vi "Pump Tags.vi"(11 "Pump Module Configs":T1[](array[typedef]) {"Settings"."ASIA Pump C"."channel" min=0 max=1 step=1; "Settings"."Masterflex"."Pump Number" min=1.0 max=20.0 step=1.0; "Settings"."Ismatech"."Pump Number" min=1.0 max=20.0 step=1.0}) -> (1 "Pump Module Tag Names":T13, 2 "All Boolean Tags 3":string[](array[string]), 3 "All  Numeric Tags 3":string[](array[string]), 4 "Pump Module Tags Array":T13[](array[typedef]))   [LabVIEW 2018]
uses:
  Pump Module Folder/Pump Module Tag Names Cluster.ctl
  Pump Module Folder/Pump Module Config Cluster.ctl
  <vilib>/Utility/miscctls.llb/LVPoint32TypeDef.ctl
  Pump Module Folder/Pump Module Settings Cluster.ctl
  Ismatec ISM 831C/Controls/Ismatech Settings Cluster.ctl
  Masterflex 7550-30/Controls/Settings Cluster.ctl
  VICI M50 Party Mode/Settings Cluster.ctl
  Measure Instrument/PID 2 Output Enum.ctl
  Tacmina QI/Tacmina QI DAQ Setting.ctl
  KNF Pump/Settings Cluster plus SIMDOS.ctl
  ASIA Pump/Pump Settings.ctl
  FLOM Pump/Settings Cluster.ctl
  SSI PR Class/SSI PR Settings Cluster.ctl
  Pump Module Folder/Pump Module.lvlib
  Ismatec ISM 831C/Ismatec ISM 831C.lvlib
  Masterflex 7550-30/Masterflex 7550-30.lvlib
  VICI M50 Party Mode/VICI M6 M50 Party Mode.lvlib
  Tacmina QI/Tacmina QI.lvlib
  KNF Pump/KNF SIMDOS.lvlib
  ASIA Pump.lvlib
  FLOM Pump/FLOM Pump.lvlib
  SSI PR Class/SSI PR Pump.lvlib
panel:
  # "Output Instruments"
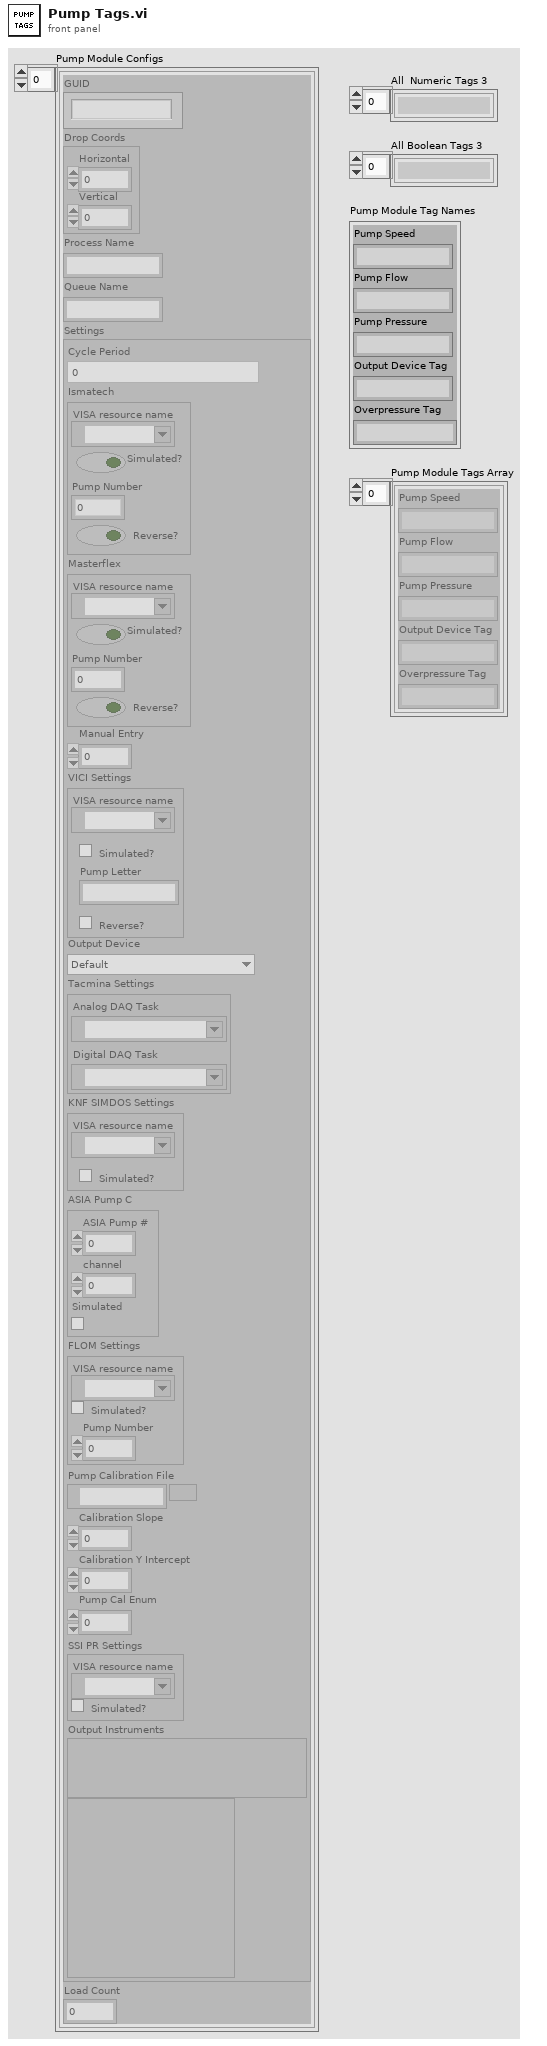
[diagram p1: front panel]
types:
  T1 = typedef "Pump Module.lvlib/Pump Module Config Cluster.ctl" = cluster{"GUID":string, "Drop Coords":T2, "Process Name":string, "Queue Name":string, "Settings":T3, "Load Count":i32}
  T2 = typedef "LVPoint32TypeDef.ctl" = cluster{"Horizontal":i32, "Vertical":i32}
  T3 = typedef "Pump Module.lvlib/Pump Module Settings Cluster.ctl" = cluster{"Cycle Period":dbl, "Ismatech":T4, "Masterflex":T5, "Manual Entry":dbl, "VICI Settings":T6, "Output Device":T7, "Tacmina Settings":T8, "KNF SIMDOS Settings":T9, "ASIA Pump C":T10, "FLOM Settings":T11, "Pump Calibration File":path, "Calibration Slope":dbl, "Calibration Y Intercept":dbl, "Pump Cal Enum":u16, "SSI PR Settings":T12}
  T4 = typedef "Ismatec ISM 831C.lvlib/Ismatech Settings Cluster.ctl" = cluster{"VISA resource name":refnum<visa-resource-name>, "Simulated?":bool, "Pump Number":dbl, "Reverse?":bool}
  T5 = typedef "Masterflex 7550-30.lvlib/Settings Cluster.ctl" = cluster{"VISA resource name":refnum<visa-resource-name>, "Simulated?":bool, "Pump Number":dbl, "Reverse?":bool}
  T6 = typedef "VICI M6 M50 Party Mode.lvlib/Settings Cluster.ctl" = cluster{"VISA resource name":refnum<visa-resource-name>, "Simulated?":bool, "Pump Letter":string, "Reverse?":bool}
  T7 = typedef "PID 2 Output Enum.ctl" = enum16{"Default", "Ismatec ISM 831C", "Masterflex 7550-30", "VICI", "Tacmina QI", "KNF SIMDOS", "ASIA Type C", "FLOM UI-22-11", "SSI PR"}
  T8 = typedef "Tacmina QI.lvlib/Tacmina QI DAQ Setting.ctl" = cluster{"Analog DAQ Task":refnum<k21>, "Digital DAQ Task":refnum<k21>}
  T9 = typedef "KNF SIMDOS.lvlib/Settings Cluster plus SIMDOS.ctl" = cluster{"VISA resource name":refnum<visa-resource-name>, "Simulated?":bool}
  T10 = typedef "ASIA Pump.lvlib/Pump Settings.ctl" = cluster{"ASIA Pump #":i32, "channel":i32, "Simulated":bool}
  T11 = typedef "FLOM Pump.lvlib/Settings Cluster.ctl" = cluster{"VISA resource name":refnum<visa-resource-name>, "Simulated?":bool, "Pump Number":dbl}
  T12 = typedef "SSI PR Pump.lvlib/SSI PR Settings Cluster.ctl" = cluster{"VISA resource name":refnum<visa-resource-name>, "Simulated?":bool}
  T13 = typedef "Pump Module.lvlib/Pump Module Tag Names Cluster.ctl" = cluster{"Pump Speed":string, "Pump Flow":string, "Pump Pressure":string, "Output Device Tag":string, "Overpressure Tag":string}
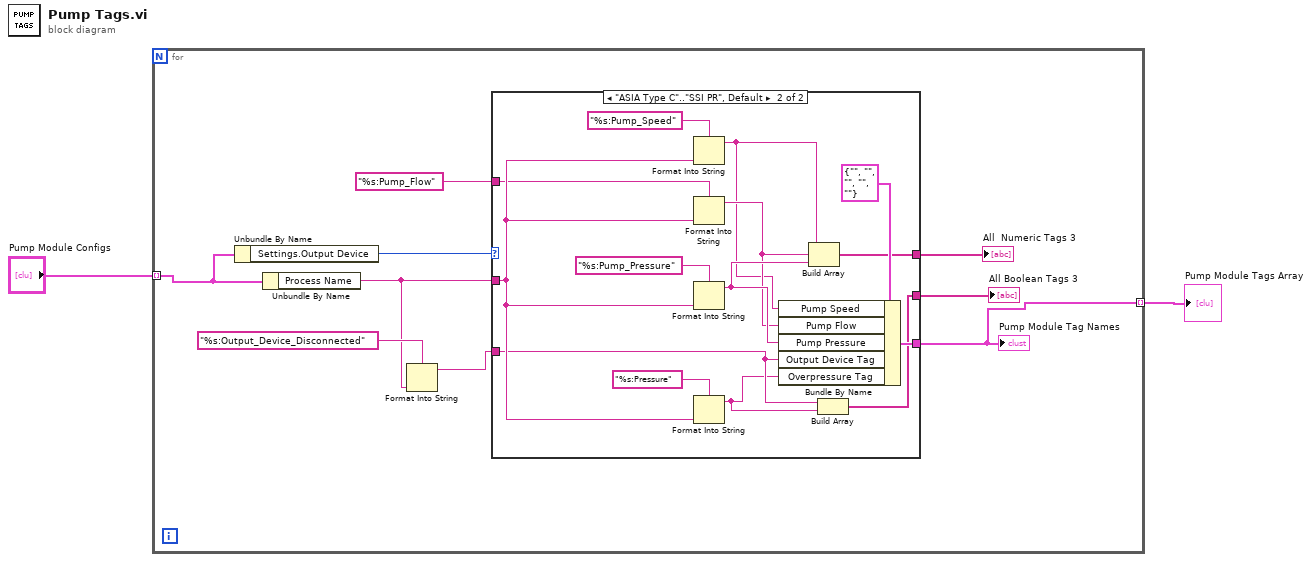
[diagram p0: block diagram]
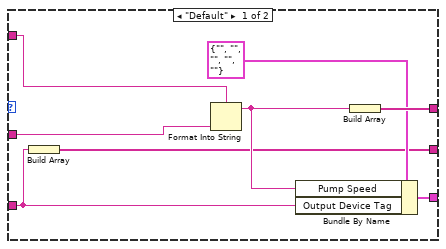
[diagram p2: hidden frame]
diagram:
  n1 = for {
    tunnel: "Pump Module Configs" -> [w4] mode=indexing
    tunnel: [w3] -> w1 mode=indexing
    n2 = Unbundle By Name(w4) -> ("Settings.Output Device"=w10:T7)
    n3 = Unbundle By Name(w4) -> ("Process Name"=w8:string)
    n4 = Format Into String(format string="%s:Output_Device_Disconnected", w8) -> (resulting string=w6:string)  [unwired: 2 in, 1 out]
    n5 = case shown="\"ASIA Type C\"..\"SSI PR\", Default" w10 {
      tunnel: w8 -> [w18 w24]
      tunnel: w6 -> [w14 w23]
      tunnel: [w19 w28] -> w9
      tunnel: [w16 w27] -> w3
      tunnel: [w13 w22] -> w7
      tunnel: "%s:Pump_Flow" ("format string") -> [w12 w20]
      frame "Default" {
        n6 = Build Array(w14) -> (w13:string[])
        n7 = Format Into String(format string=w12, w18) -> (resulting string=w17:string)  [unwired: 2 in, 1 out]
        n8 = Bundle By Name(cluster=T13 {"Pump Speed"="", "Pump Flow"="", "Pump Pressure"="", "Output Device Tag"="", "Overpressure Tag"=""} ("Feed Module Tag Names"), "Pump Speed"=w17, "Output Device Tag"=w14) -> (w16:T13)
        n9 = Build Array(w17) -> (w19:string[])
      }
      frame "ASIA Type C".."SSI PR", Default {
        n10 = Format Into String(format string="%s:Pump_Speed", w24) -> (resulting string=w26:string)  [unwired: 2 in, 1 out]
        n11 = Format Into String(format string=w20, w24) -> (resulting string=w32:string)  [unwired: 2 in, 1 out]
        n12 = Format Into String(format string="%s:Pump_Pressure", w24) -> (resulting string=w33:string)  [unwired: 2 in, 1 out]
        n13 = Format Into String(format string="%s:Pressure", w24) -> (resulting string=w21:string)  [unwired: 2 in, 1 out]
        n14 = Bundle By Name(cluster=T13 {"Pump Speed"="", "Pump Flow"="", "Pump Pressure"="", "Output Device Tag"="", "Overpressure Tag"=""} ("Feed Module Tag Names"), "Pump Speed"=w26, "Pump Flow"=w32, "Pump Pressure"=w33, "Output Device Tag"=w23, "Overpressure Tag"=w21) -> (w27:T13)
        n15 = Build Array(w26, w32, w33) -> (w28:string[])
        n16 = Build Array(w23, w21) -> (w22:string[])
      }
    }
    "Pump Module Tag Names" <- w3
    "All Boolean Tags 3" <- w7
    "All  Numeric Tags 3" <- w9
  }
  "Pump Module Tags Array" <- w1
